vi "Lab Panel V5.12.vi"() -> ()   [LabVIEW 2013] (continued)
            n3271 = local read "SET LAB05-2"() -> (w5932:T5)
            n3272 = local read "SET LAB05-1"() -> (w5933:T5)
            n3273 = local read "SET LAB04-1"() -> (w5935:T5)
            n3274 = local read "SET LAB04-2"() -> (w5934:T5)
            n3275 = local read "SET LAB03-1"() -> (w5937:T5)
            n3276 = local read "SET LAB03-2"() -> (w5936:T5)
            n3277 = local read "SET LAB02-2"() -> (w5938:T5)
            n3278 = local read "SET LAB01-2"() -> (w5940:T5)
            n3279 = local read "SET LAB02-1"() -> (w5939:T5)
            n3280 = local read "SET LAB01-1"() -> (w5941:T5)
            n3281 = global write "Global display 2.vi" "SET LAB05-2"(w5932) -> ()
            n3282 = global write "Global display 2.vi" "SET LAB05-1"(w5933) -> ()
            n3283 = global write "Global display 2.vi" "SET LAB04-1"(w5935) -> ()
            n3284 = global write "Global display 2.vi" "SET LAB04-2"(w5934) -> ()
            n3285 = global write "Global display 2.vi" "SET LAB03-2"(w5936) -> ()
            n3286 = global write "Global display 2.vi" "SET LAB02-2"(w5938) -> ()
            n3287 = global write "Global display 2.vi" "SET LAB03-1"(w5937) -> ()
            n3288 = global write "Global display 2.vi" "SET LAB01-2"(w5940) -> ()
            n3289 = global write "Global display 2.vi" "SET LAB01-1"(w5941) -> ()
            n3290 = global write "Global display 2.vi" "SET LAB02-1"(w5939) -> ()
            n3291 = local read "RESULT LAB01-1"() -> (w5931:bool)
            n3292 = local read "RESULT LAB03-2"() -> (w5926:bool)
            n3293 = local read "RESULT LAB04-1"() -> (w5925:bool)
            n3294 = local read "RESULT LAB04-2"() -> (w5924:bool)
            n3295 = local read "RESULT LAB02-2"() -> (w5928:bool)
            n3296 = local read "RESULT LAB01-2"() -> (w5930:bool)
            n3297 = local read "RESULT LAB02-1"() -> (w5929:bool)
            n3298 = local read "RESULT LAB03-1"() -> (w5927:bool)
            n3299 = local read "RESULT LAB05-1"() -> (w5923:bool)
            n3300 = local read "RESULT LAB05-2"() -> (w5922:bool)
            n3301 = global write "Global display 2.vi" "RESULT LAB05-1"(w5923) -> ()
            n3302 = global write "Global display 2.vi" "RESULT LAB01-2"(w5930) -> ()
            n3303 = global write "Global display 2.vi" "RESULT LAB03-2"(w5926) -> ()
            n3304 = global write "Global display 2.vi" "RESULT LAB04-1"(w5925) -> ()
            n3305 = global write "Global display 2.vi" "RESULT LAB04-2"(w5924) -> ()
            n3306 = global write "Global display 2.vi" "RESULT LAB05-2"(w5922) -> ()
            n3307 = global write "Global display 2.vi" "RESULT LAB03-1"(w5927) -> ()
            n3308 = global write "Global display 2.vi" "RESULT LAB02-1"(w5929) -> ()
            n3309 = global write "Global display 2.vi" "RESULT LAB02-2"(w5928) -> ()
            n3310 = global write "Global display 2.vi" "RESULT LAB01-1"(w5931) -> ()
          }
          frame #21 {
            # "simulate values"
            n3311 = global write "Global display 4.vi" "LAB deg C"("LAB deg C") -> ()
          }
          frame #22 {
            # "end main and display program"
            n3312 = Quit LabVIEW(quit? (T)="stop all") -> ()
            n3313 = global write "Global display 1.vi" "stop disp"("stop all") -> ()
          }
        }
        n3314 = node-c288() -> ()  [unwired: 1 in, 1 out]
        "loops" <- w315
      }
      n3315 = node-c288(w288) -> ()  [unwired: 1 out]
    }
  }
